vi "Counter - Read Encoder Velocity5 (Continuous Clock).vi"() -> ()   [LabVIEW 2015]
doc: "This example demonstrates how to use a counter input along with an external clock to continually sample the angular velocity measured from an encoder.\n\nFor instructions on how to connect your signals to the DAQ device, refer to your device documentation."
uses:
  <vilib>/Utility/error.llb/DialogType.ctl
  <vilib>/DAQmx/read.llb/DAQmx Read (Analog 1D Wfm NChan NSamp).vi
  <vilib>/DAQmx/read.llb/DAQmx Read (Counter 2D DBL NChan NSamp).vi
  <vilib>/DAQmx/create/channels.llb/DAQmx Create Channel (CI-Velocity-Linear).vi
  <vilib>/DAQmx/create/channels.llb/DAQmx Create Channel (AI-Voltage-Basic).vi
  <vilib>/DAQmx/configure/timing.llb/DAQmx Timing (Sample Clock).vi
  <vilib>/DAQmx/miscellaneous.llb/DAQmx Fill In Error Info.vi
  <resource>/objmgr/daqmx.rc
panel:
  in  "Channel 2":bool=TRUE
  in  "Channel 1":bool=TRUE
  out "appended path":path
  in  "Row 1 Header":string="Header Information Row 1"
  out "Boolean":bool
  out "Waveform Chart":dbl(graph)
  out "Numeric Indicator":dbl format="%.1g"
  in  "Counter 0":tag="Mantis1_1Mod4/ctr0"
  in  "B Input Terminal":tag="/Mantis1_1Mod4/PFI7"
  in  "A Input Terminal":tag="/Mantis1_1Mod4/PFI0"
  in  "Stop":bool
  in  "Samples per Loop":i32=1
  in  "Sample Rate":dbl=100.0
  in  "Sample Clock Source":tag="OnboardClock"
  # "MPH"
  # "Channel Settings"
  # "Saving data"
  # "Timing Settings"
  # "Trigger Rising Edge?"
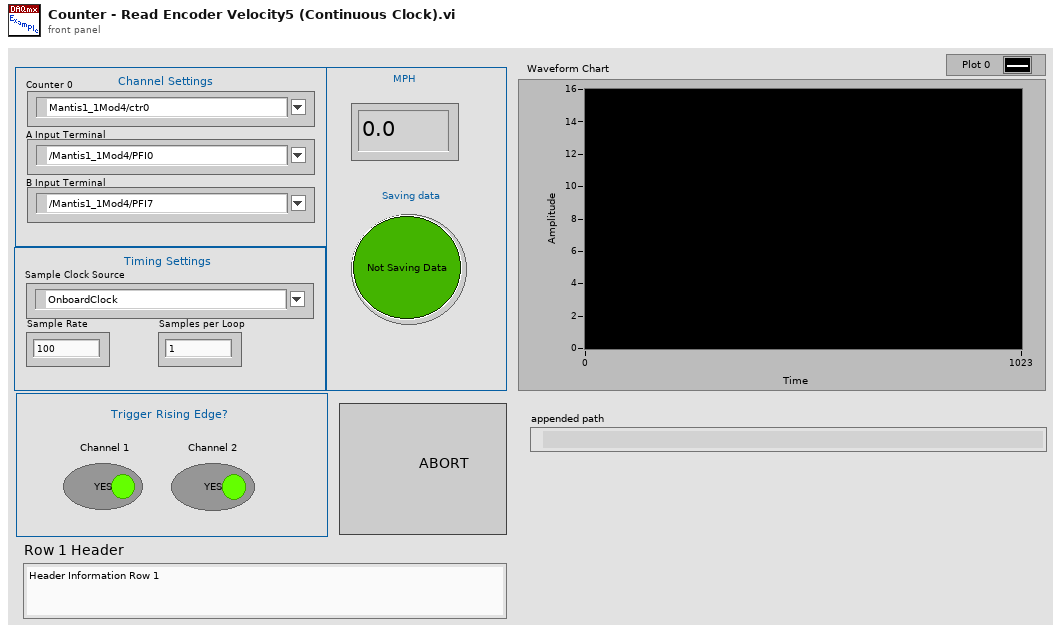
[diagram p1: front panel]
types:
  T1 = typedef "DialogType.ctl" = u16
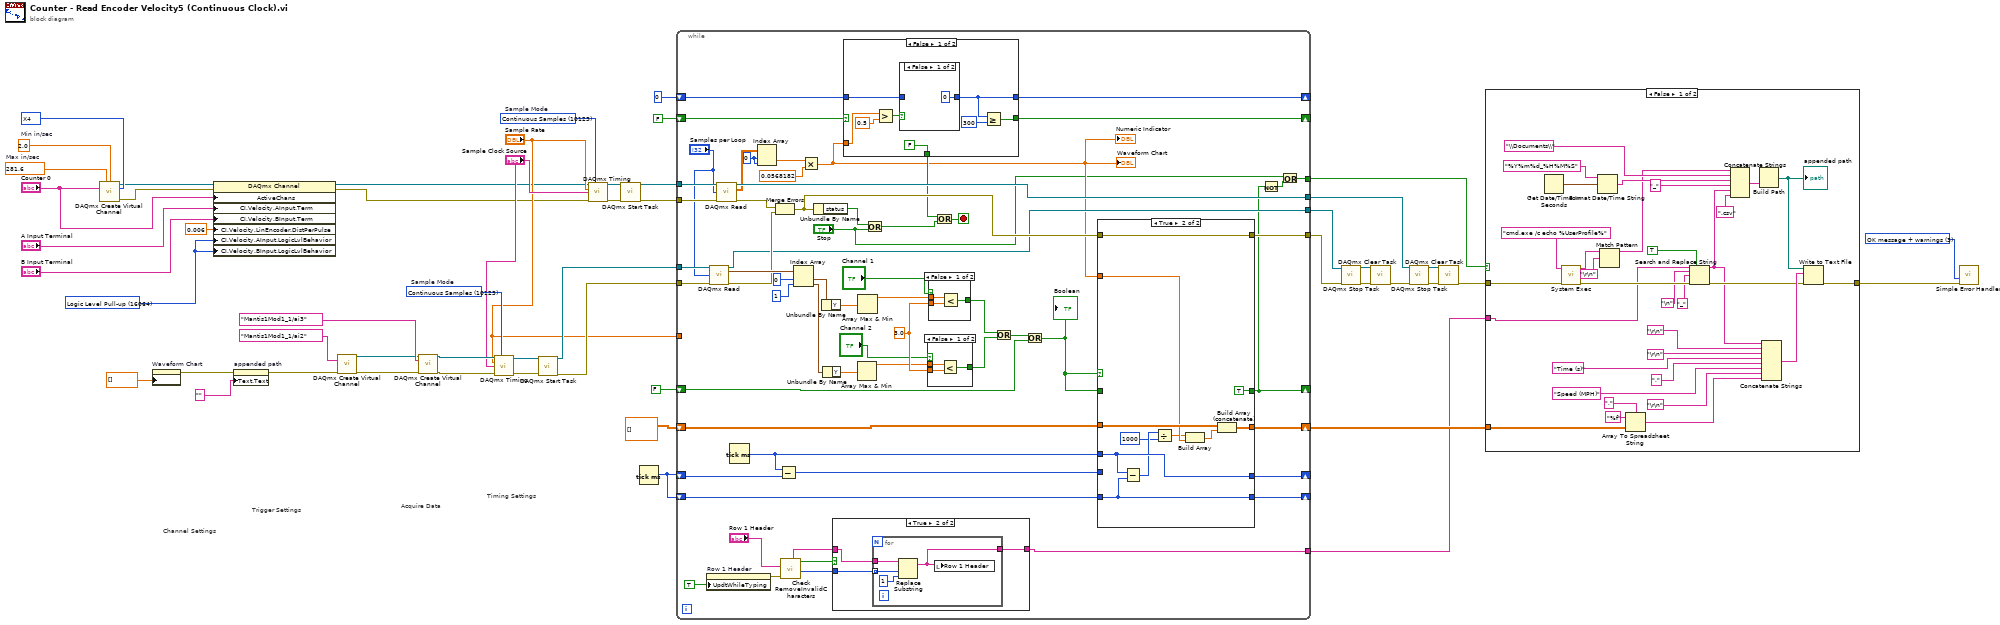
[diagram p0: block diagram]
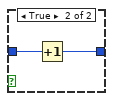
[diagram p3: hidden frame]
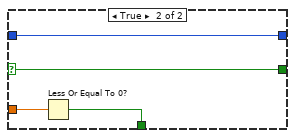
[diagram p4: hidden frame]
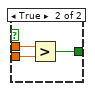
[diagram p6: hidden frame]
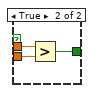
[diagram p7: hidden frame]
diagram:
  w5 = 16064 items=["Logic Level Pull-up"=16064, "None"=10230] ("CI.Velocity.AInput.LogicLvlBehavior")
  w34 = 10123 items=["Finite Samples"=10178, "Continuous Samples"=10123, "Hardware Timed Single Point"=12522]  # Sample Mode
  w47 = 281.6  # Max in/sec
  w46 = 2.0  # Min in/sec
  w41 = 10092 items=["X1"=10090, "X2"=10091, "X4"=10092, "Two Pulse Counting"=10313] ("decoding type")
  w48 = T1 3 items=["no dialog", "OK message", "continue or stop message", "OK message + warnings", "continue/stop + warnings"] ("type of dialog (OK msg:1)")
  w53 = 10123 items=["Finite Samples"=10178, "Continuous Samples"=10123, "Hardware Timed Single Point"=12522]  # Sample Mode
  # "Acquire Data"
  # "Trigger Settings"
  # "Timing Settings"
  # "Channel Settings"
  n1 = call-poly <vilib>:"DAQmx Create Virtual Channel.vi"("maximum value"=w47, "minimum value"=w46, "counter"="Counter 0", "decoding type"=w41) -> ("task out"=w9:refnum<k21>, "error out"=w8:errorcluster)  [unwired: 10 in]
  n2 = property on="Waveform Chart" class="WFChart (strict)"("History Data"=dbl[] []) -> (error out=w19:errorcluster)  [unwired: 2 in, 1 out]
  n3 = property class="DAQmx Channel"(reference=w9, error in=w8, "ActiveChans"="Counter 0", "CI.Velocity.AInput.Term"="A Input Terminal", "CI.Velocity.BInput.Term"="B Input Terminal", "CI.Velocity.LinEncoder.DistPerPulse"=0.006, "CI.Velocity.AInput.LogicLvlBehavior"=w5, "CI.Velocity.BInput.LogicLvlBehavior"=w5) -> (reference out=w6:refnum<k21>, error out=w7:errorcluster)
  n4 = property on="appended path" class="Path"(error in=w19, "Text.Text"="" ("Path Text.Text")) -> (error out=w18:errorcluster)  [unwired: 1 in, 1 out]
  n5 = call-poly <vilib>:"DAQmx Create Virtual Channel.vi"("physical channels"=tag "Mantis1Mod1_1/ai2", "error in"=w18) -> ("task out"=w38:refnum<k21>, "error out"=w37:errorcluster)  [unwired: 12 in]
  n6 = call-poly <vilib>:"DAQmx Create Virtual Channel.vi"("task in"=w38, "physical channels"=tag "Mantis1Mod1_1/ai3", "error in"=w37) -> ("task out"=w33:refnum<k21>, "error out"=w32:errorcluster)  [unwired: 11 in]
  n7 = call-poly <vilib>:"DAQmx Timing.vi"("task/channels in"=w33, "sample mode"=w34, "rate"="Sample Rate", "source"="Sample Clock Source", "error in"=w32) -> ("task out"=w30:refnum<k21>, "error out"=w29:errorcluster)  [unwired: 9 in]
  n8 = call <vilib>:"DAQmx Start Task.vi"("task/channels in"=w30, "error in"=w29) -> ("task out"=w27:refnum<k21>, "error out"=w26:errorcluster)  [unwired: 12 in]
  n9 = call-poly <vilib>:"DAQmx Timing.vi"("task/channels in"=w6, "sample mode"=w53, "rate"="Sample Rate", "source"="Sample Clock Source", "error in"=w7) -> ("task out"=w35:refnum<k21>, "error out"=w36:errorcluster)  [unwired: 9 in]
  n10 = call <vilib>:"DAQmx Start Task.vi"("task/channels in"=w35, "error in"=w36) -> ("task out"=w52:refnum<k21>, "error out"=w51:errorcluster)  [unwired: 12 in]
  n11 = Tick Count (ms)() -> (millisecond timer value=w20:u32)
  n12 = while {
    tunnel: w52 -> [w113]
    tunnel: w51 -> [w112]
    tunnel: [w111] -> w13
    tunnel: w27 -> [w95]
    tunnel: w26 -> [w94]
    tunnel: "Sample Rate" -> [_]
    shift-right: [w88] -> _
    shift-left: w20 -> [w87]
    shift-right: [w80] -> _
    shift-left: w20 -> [w81]
    shift-right: [w78] -> w23
    shift-left: dbl[][] [] -> [w79]
    tunnel: [w77] -> w11
    tunnel: [w74] -> w12
    tunnel: [w57] -> w10
    shift-right: [w58] -> _
    shift-left: FALSE -> [w72]
    tunnel: [w64] -> w3
    shift-right: [w61] -> _
    shift-left: FALSE -> [w63]
    shift-right: [w54] -> _
    shift-left: 0 -> [w55]
    stop <- w92 stop-if-true
    w104 = 3.0 ("y")
    w91 = 0 ("disabled index (col)")
    n13 = property on="Row 1 Header" class="Str"("UpdtWhileTyping"=TRUE ("Update While Typing?")) -> (error out=w68:errorcluster)  [unwired: 2 in, 1 out]
    n14 = call-poly <vilib>:"DAQmx Read.vi"("task/channels in"=w95, "number of samples per channel"="Samples per Loop", "error in"=w94) -> ("task out"=w74:refnum<k21>, "data"=w107:waveform(dbl)[], "error out"=w85:errorcluster)  [unwired: 10 in]
    n15 = call-poly <vilib>:"DAQmx Read.vi"("task/channels in"=w113, "number of samples per channel"="Samples per Loop", "error in"=w112) -> ("task out"=w111:refnum<k21>, "data"=w109:dbl[][], "error out"=w84:errorcluster)  [unwired: 10 in]
    n16 = Tick Count (ms)() -> (millisecond timer value=w86:u32)
    n17 = Index Array(array=w109, index (row)=w91, index (col)=w91) -> (element=w90:dbl)
    n18 = Merge Errors(w84, w85) -> (w83:errorcluster)
    n19 = Subtract(x=w86, y=w87) -> (x-y=w82:u32)
    n20 = call "Check RemoveInvalidCharacters.vi"("error in"=w68, "Path String"="Row 1 Header") -> ("Offset to Bad Character(s)"=w65:i32[], "Bad Filename?"=w67:bool, "Path String Out"=w66:string)  [unwired: 5 in, 2 out]
    n21 = Index Array(array=w107, index #1=0 ("index"), index #2=1 ("index")) -> (element #1=w97:waveform(dbl), element #2=w100:waveform(dbl))
    n22 = Multiply(x=w90, y=0.0568182) -> (x*y=w60:dbl)
    "Numeric Indicator" <- w60
    "Waveform Chart" <- w60
    n23 = Unbundle By Name(w83) -> ("status"=w110:bool)
    n24 = Unbundle By Name(w97) -> ("Y"=w98:dbl[])
    n25 = Unbundle By Name(w100) -> ("Y"=w101:dbl[])
    n26 = case shown="True" w67 {
      tunnel: w66 -> [w129 w131]
      tunnel: w65 -> [_ w132]
      tunnel: [w129 w130] -> w64
      frame False {
      }
      frame True {
        n27 = for {
          tunnel: w132 -> [w136] mode=indexing
          tunnel: w131 -> [w135]
          tunnel: [w133] -> w130
          n28 = Replace Substring(2:1 ("length (len. of substring)"), 3:w136, 5:w135) -> (1:w133:string)  [unwired: 1 in, 1 out]
          n29 = local write "Row 1 Header"(w133) -> ()
        }
      }
    }
    n30 = case shown="False" w63 {
      selector: w63 -> [_ w126]
      tunnel: w60 -> [w119 w128]
      tunnel: [FALSE w127] -> w62
      tunnel: [w114 w126] -> w61
      tunnel: w55 -> [w117 w125]
      tunnel: [w116 w125] -> w54
      frame False {
        n31 = Greater?(x=w119, y=0.5) -> (0:w120:bool)
        n32 = case shown="False" w120 {
          tunnel: w117 -> [_ w124]
          tunnel: [0 w123] -> w116
          frame False {
          }
          frame True {
            n33 = Increment(x=w124) -> (x+1=w123:i32)
          }
        }
        n34 = Greater Or Equal?(x=w116, y=300) -> (x >= y?=w114:bool)
      }
      frame True {
        n35 = Less Or Equal To 0?(x=w128) -> (x <= 0?=w127:bool)
      }
    }
    n36 = Array Max & Min(array=w101) -> (max value=w103:dbl)  [unwired: 3 out]
    n37 = Array Max & Min(array=w98) -> (max value=w102:dbl)  [unwired: 3 out]
    n38 = Or(x=w110, y="Stop") -> (x .or. y?=w93:bool)
    n39 = case shown="False" "Channel 2" {
      tunnel: [w138 w142] -> w106
      tunnel: w104 -> [w139 w141]
      tunnel: w103 -> [w137 w140]
      frame False {
        n40 = Less?(x=w137, y=w139) -> (x < y?=w138:bool)
      }
      frame True {
        n41 = Greater?(x=w140, y=w141) -> (0:w142:bool)
      }
    }
    n42 = case shown="False" "Channel 1" {
      tunnel: [w145 w148] -> w105
      tunnel: w104 -> [w143 w147]
      tunnel: w102 -> [w144 w146]
      frame False {
        n43 = Less?(x=w144, y=w143) -> (x < y?=w145:bool)
      }
      frame True {
        n44 = Greater?(x=w146, y=w147) -> (0:w148:bool)
      }
    }
    n45 = Or(x=w62, y=w93) -> (x .or. y?=w92:bool)
    n46 = Or(x=w105, y=w106) -> (x .or. y?=w73:bool)
    n47 = Or(x=w73, y=w72) -> (x .or. y?=w71:bool)
    "Boolean" <- w71
    n48 = case shown="True" w71 {
      tunnel: w60 -> [_ w160]
      tunnel: w86 -> [w150 w158]
      tunnel: [w150 w158] -> w88
      tunnel: w83 -> [w151 w159]
      tunnel: w82 -> [_ _]
      tunnel: w81 -> [_ w157]
      tunnel: [w150 w157] -> w80
      tunnel: [w152 w162] -> w78
      tunnel: w79 -> [w152 w163]
      tunnel: [w151 w159] -> w77
      tunnel: [w149 TRUE] -> w58
      tunnel: w71 -> [w149 _]
      frame False {
      }
      frame True {
        n49 = Subtract(x=w158, y=w157) -> (x-y=w155:u32)
        n50 = Divide(x=w155, y=u32 1000) -> (x/y=w156:dbl)
        n51 = Build Array(w156, w160) -> (w161:dbl[])
        n52 = Build Array (concatenate)(w163, w161) -> (w162:dbl[][])
      }
    }
    n53 = Not(x=w58) -> (.not. x?=w56:bool)
    n54 = Or(x="Stop", y=w56) -> (x .or. y?=w57:bool)
  }
  n55 = call <vilib>:"DAQmx Stop Task.vi"("task/channels in"=w12, "error in"=w11) -> ("task out"=w16:refnum<k21>, "error out"=w15:errorcluster)  [unwired: 12 in]
  n56 = call <vilib>:"DAQmx Clear Task.vi"("task in"=w16, "error in"=w15) -> ("error out"=w14:errorcluster)  [unwired: 13 in]
  n57 = call <vilib>:"DAQmx Stop Task.vi"("task/channels in"=w13, "error in"=w14) -> ("task out"=w49:refnum<k21>, "error out"=w50:errorcluster)  [unwired: 12 in]
  n58 = call <vilib>:"DAQmx Clear Task.vi"("task in"=w49, "error in"=w50) -> ("error out"=w21:errorcluster)  [unwired: 13 in]
  n59 = case shown="False" w10 {
    tunnel: w23 -> [w190 _]
    tunnel: [w186 w196] -> w22
    tunnel: w21 -> [w176 w196]
    tunnel: w3 -> [w164 _]
    frame False {
      n60 = Get Date/Time In Seconds() -> (seconds since 1Jan1904=w184:timestamp)
      n61 = call <vilib>:"System Exec.vi"("error in (no error)"=w176, "command line"="cmd.exe /c echo %UserProfile%") -> ("error out"=w170:errorcluster, "standard output"=w175:string)  [unwired: 6 in, 2 out]
      n62 = Format Date/Time String(time format string (%c)="%Y%m%d_%H%M%S", seconds (now)=w184) -> (date/time string=w182:string)  [unwired: 1 out]
      n63 = Match Pattern(string=w175, regular expression="\r\n") -> (before substring=w174:string)  [unwired: 1 in, 3 out]
      n64 = Array To Spreadsheet String(delimiter (Tab)=",", array=w190, 3:"%f" ("format string")) -> (spreadsheet string=w187:string)
      n65 = Search and Replace String(replace all?=TRUE ("replace all? (F)"), input string=w164, search string="\n", replace string="_" ("replace string (\"\")"), error in=w170) -> (result string=w168:string, error out=w169:errorcluster)  [unwired: 3 in, 2 out]
      n66 = Concatenate Strings(w174, "\\Documents\\" ("string"), w182, "_" ("string"), w168, ".csv" ("string")) -> (w181:string)
      n67 = Build Path(name or relative path=w181) -> (appended path=w180:path)  [unwired: 1 in]
      "appended path" <- w180
      n68 = Concatenate Strings(w168, "\r\n", "\r\n", "Time (s)", ",", "Speed (MPH)", "\r\n", w187) -> (w185:string)
      n69 = Write to Text File(file (use dialog)=w180, text=w185, error in=w169) -> (error out=w186:errorcluster)  [unwired: 1 in, 2 out]
    }
    frame True {
    }
  }
  n70 = call <vilib>:"Simple Error Handler.vi"("type of dialog (OK msg:1)"=w48, "error in (no error)"=w22) -> ()  [unwired: 3 in, 5 out]
